vi "SL2_AD_DLL_Phoibos_SetChannelROI.vi"(6 "pHandle":u32, 7 "error in":errorcluster, 8 "ROI_2D":u32[][](array[numeric]), 9 "chanID":u32, 10 "dll path in":path) -> (0 "error out":errorcluster, 3 "dll path out":path)   [LabVIEW 2010]
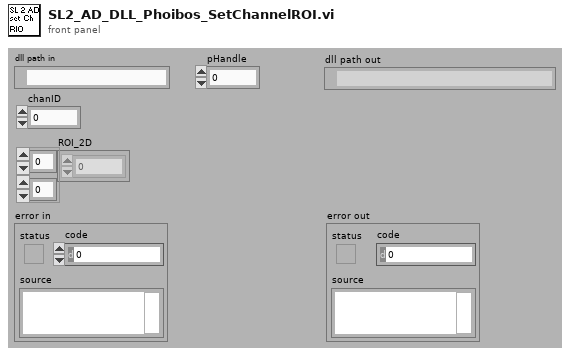
[diagram p1: front panel]
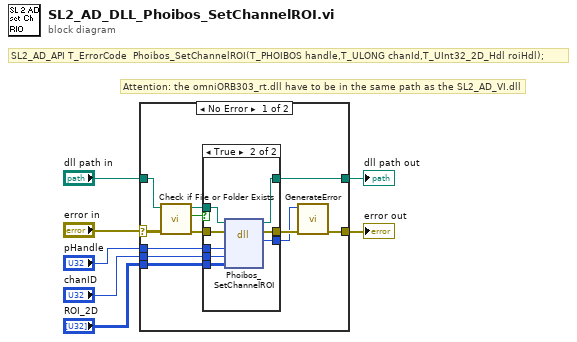
[diagram p0: block diagram]
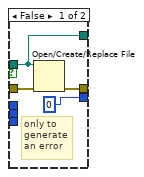
[diagram p2: hidden frame]
diagram:
  # "SL2_AD_API T_ErrorCode  Phoibos_SetChannelROI(T_PHOIBOS handle,T_ULONG chanId,T_UInt32_2D_Hdl roiHdl);"
  # "Attention: the omniORB303_rt.dll have to be in the same path as the SL2_AD_VI.dll"
  n1 = case shown="No Error" "error in" {
    selector: "error in" -> [w18 w32]
    tunnel: [w12 w32] -> w7
    tunnel: [w19 w33] -> w6
    tunnel: "dll path in" -> [w17 w33]
    tunnel: "pHandle" -> [w16 _]
    tunnel: "chanID" -> [w15 _]
    tunnel: "ROI_2D" -> [w14 _]
    frame No Error {
      n2 = call <vilib>:"Check if File or Folder Exists.vi"("error in (no error)"=w18, "path"=w17) -> ("error out"=w8:errorcluster, "file or folder exists?"=w10:bool, "dup path"=w9:path)  [unwired: 7 in]
      n3 = case shown="True" w10 {
        tunnel: [w22 w30] -> w13
        tunnel: [u32 0 ("error_code") w27] -> w11
        tunnel: [w21 w28] -> w19
        tunnel: w9 -> [w21 w29]
        tunnel: w8 -> [w23 w31]
        tunnel: w16 -> [_ w26]
        tunnel: w15 -> [_ w25]
        tunnel: w14 -> [_ w24]
        frame False {
          # "only to generate an error"
          n4 = Open/Create/Replace File(file path (use dialog)=w21, error in=w23) -> (error out=w22:errorcluster)  [unwired: 4 in, 2 out]
        }
        frame True {
          n5 = dll-call lib="C:/Programme/SPECS/SpecsLab2/programming/LabView7.1/SL2_AD_VI.dll" fn="Phoibos_SetChannelROI" ("SetVoltage")(path in=w29, error in=w31, "pHandle"=w26, "chanID"=w25, "rioHdl"=w24) -> (path out=w28:path, error out=w30:errorcluster, "error_code"=w27:u32)  [unwired: 4 in]
        }
      }
      n6 = call "GenerateError.vi"("error in"=w13, "error_code"=w11) -> ("error out"=w12:errorcluster)  [unwired: 9 in]
    }
    frame Error {
    }
  }
  "error out" <- w7
  "dll path out" <- w6
